vi "updateXYGraph.vi"(6 "reference plot":cluster{"Value":dbl[], "Value":dbl[]}, 8 "error in (no error)":errorcluster, 9 "wavelength":refnum<vi>, 10 "counts":refnum<vi>, 11 "XYGraph in":refnum<vi>) -> (0 "error out":errorcluster, 2 "output cluster":cluster{"Value":dbl[], "Value":dbl[]})   [LabVIEW 2013]
panel:
  out "XY Graph":cluster{dbl, dbl}[](graph)
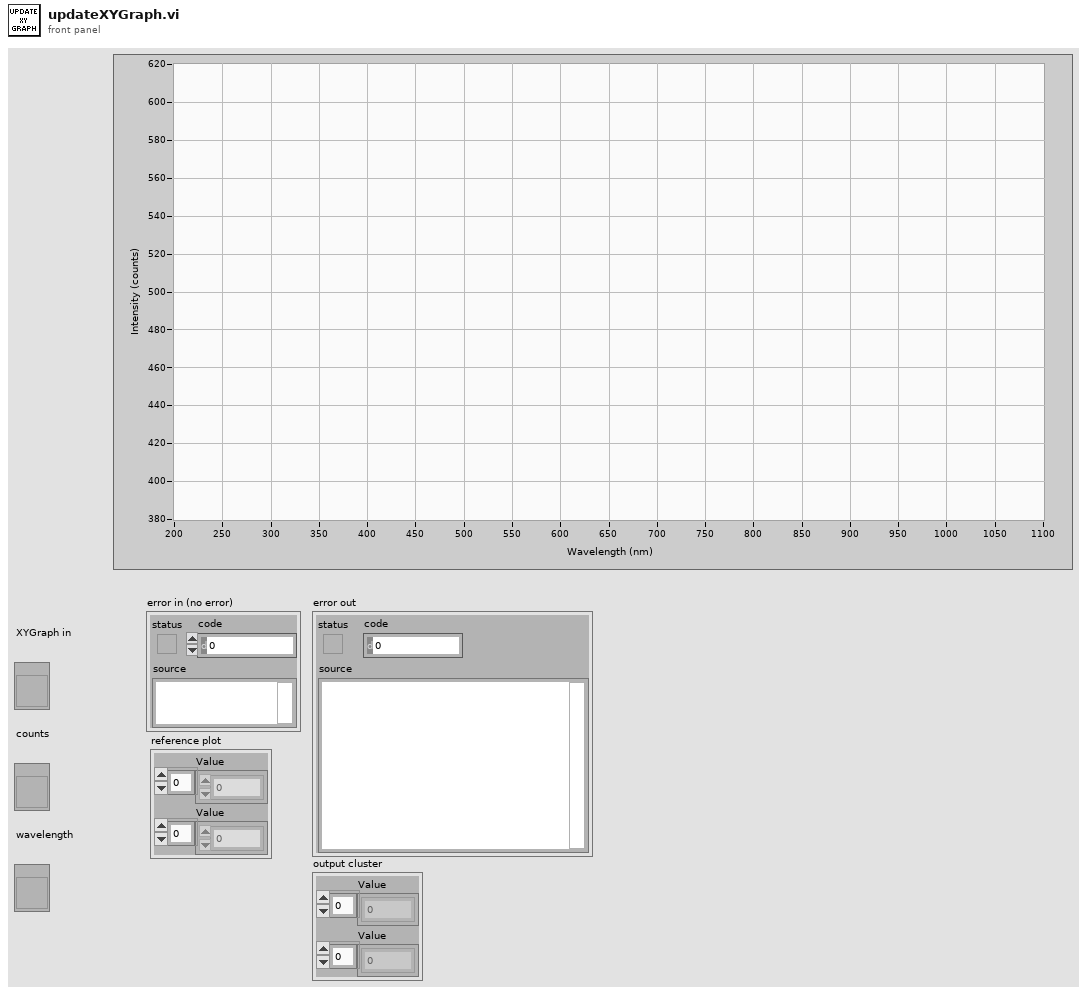
[diagram p1: front panel]
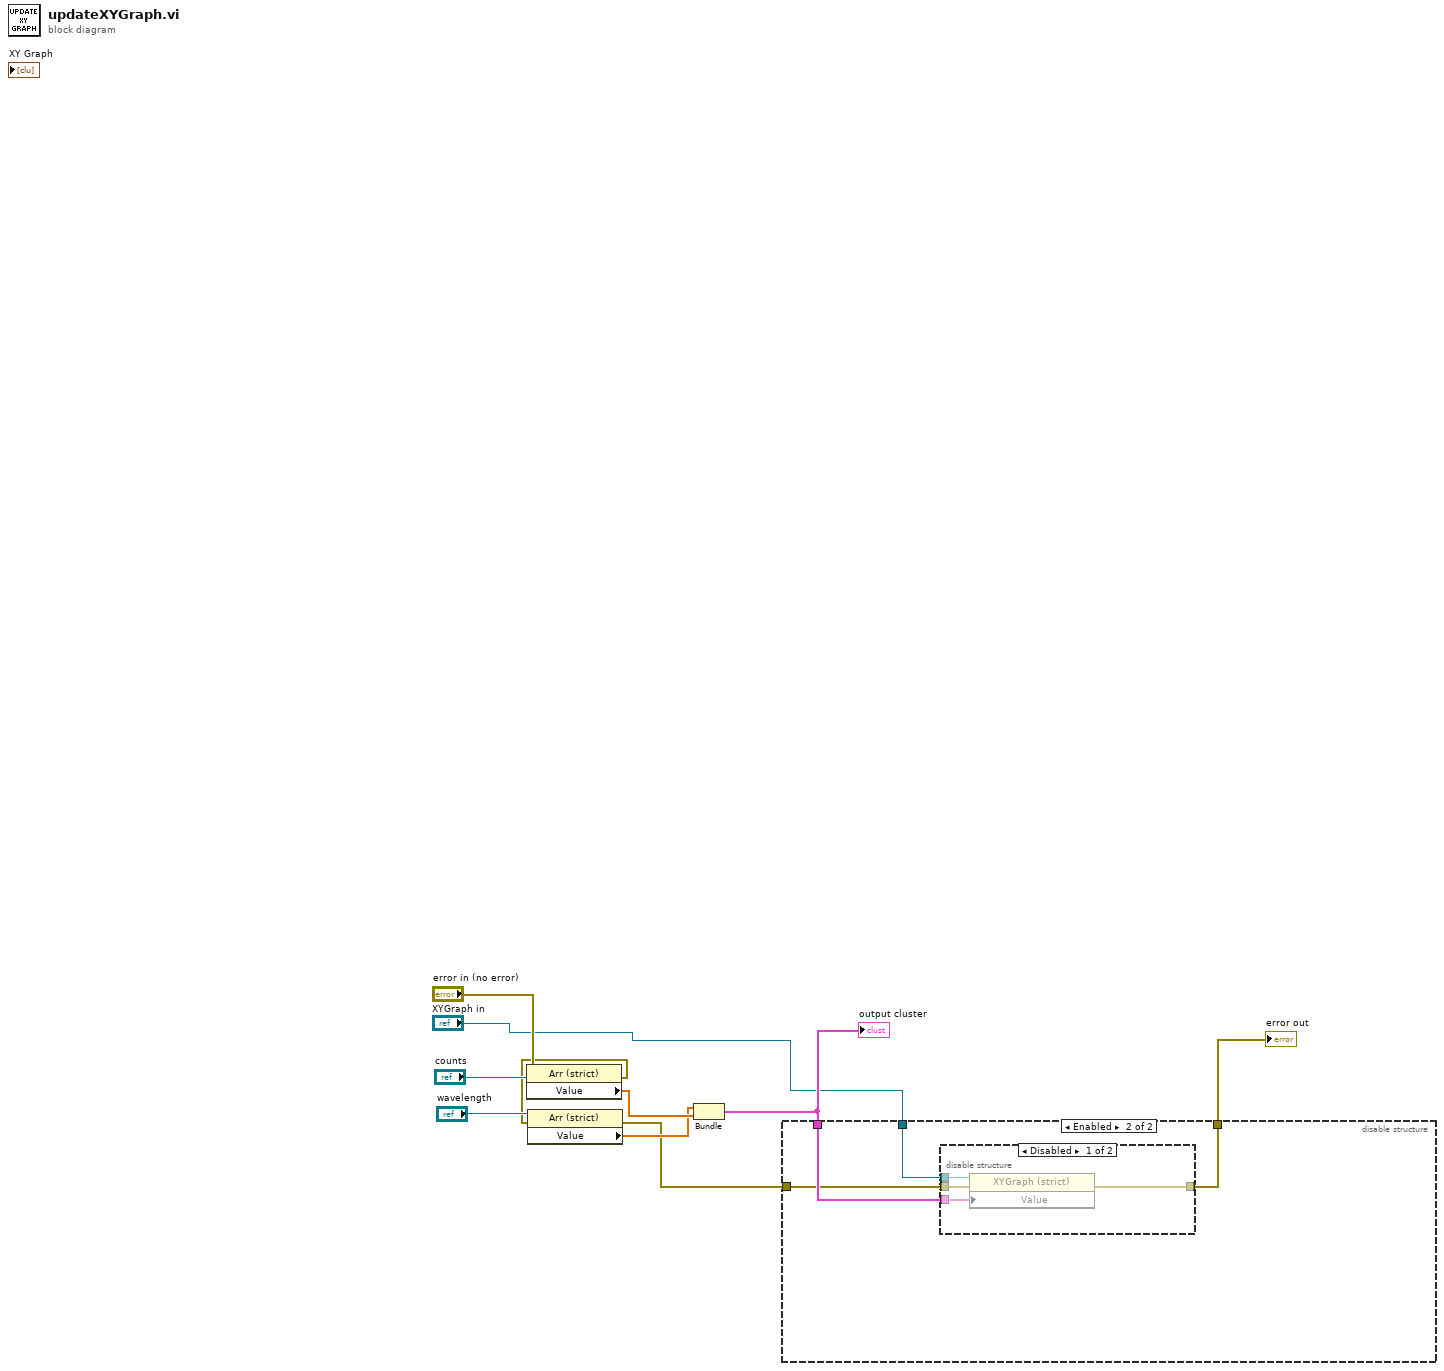
[diagram p0: block diagram]
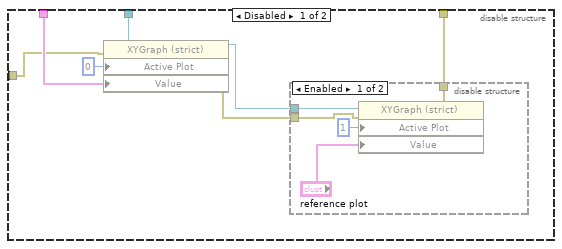
[diagram p2: hidden frame]
diagram:
  n1 = property class="Arr (strict)"(reference="counts", error in="error in (no error)") -> (error out=w5:errorcluster, "Value"=w10:dbl[])  [unwired: 1 out]
  n2 = property class="Arr (strict)"(reference="wavelength", error in=w5) -> (error out=w3:errorcluster, "Value"=w9:dbl[])  [unwired: 1 out]
  n3 = Bundle("Value"=w9, "Value"=w10) -> (w4:cluster{"Value":dbl[], "Value":dbl[]})  [unwired: 1 in]
  "output cluster" <- w4
  n4 = disable-structure shown="Enabled" {
    disable-tunnel: "XYGraph in" -> [w17 w27]
    disable-tunnel: w4 -> [w15 w26]
    disable-tunnel: w3 -> [w12 w25]
    disable-tunnel: [w11 w24] -> w2
    frame Disabled {
      n5 = property class="XYGraph (strict)"(reference=w17, error in=w12, "Active Plot"=u32 0, "Value"=w15) -> (reference out=w14:refnum<vi>, error out=w13:errorcluster)
      n6 = disable-structure shown="Enabled" {
        disable-tunnel: w14 -> [w22 _]
        disable-tunnel: w13 -> [w19 w23]
        disable-tunnel: [w18 w23] -> w11
        frame Enabled {
          n7 = property class="XYGraph (strict)"(reference=w22, error in=w19, "Active Plot"=u32 1, "Value"="reference plot") -> (error out=w18:errorcluster)  [unwired: 1 out]
        }
        frame Disabled {
        }
      }
    }
    frame Enabled {
      n8 = disable-structure shown="Disabled" {
        disable-tunnel: w27 -> [w31 _]
        disable-tunnel: w26 -> [w30 _]
        disable-tunnel: w25 -> [w29 _]
        disable-tunnel: [w28 _] -> w24
        frame Disabled {
          n9 = property class="XYGraph (strict)"(reference=w31, error in=w29, "Value"=w30) -> (error out=w28:errorcluster)  [unwired: 1 out]
        }
        frame Enabled {
        }
      }
    }
  }
  "error out" <- w2
